vi "Setup Path.vi"(0 "Path in":refnum<class "Path.lvclass">, 5 "TSM Context":T1, 7 "Path Callback References in":refnum<vi>[](array[refnum]), 11 "error in":errorcluster) -> (4 "Path out":refnum<class "Path.lvclass">, 15 "error out":errorcluster)   [LabVIEW 2023, in "RFFixtureCharact.Public.lvlib"]
uses:
  RFFixtureCharact.Public.lvlib
  Common/Base Classes/Path/Path.lvclass
  <vilib>/NI_TestStand_SemiconductorModule/NI_TestStand_Semiconductor_Module.lvlibp/PinMap/General/SemiconductorModuleContext.ctl
  Common/RFCalAndFixtureCharact.Common.lvlib
  <vilib>/NI_TestStand_SemiconductorModule/NI_TestStand_Semiconductor_Module.lvlibp
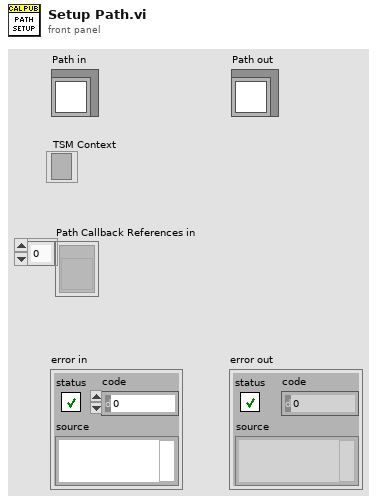
[diagram p1: front panel]
types:
  T1 = typedef "NI_TestStand_Semiconductor_Module.lvlibp/SemiconductorModuleContext.ctl" = refnum<k7>
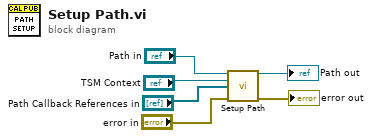
[diagram p0: block diagram]
diagram:
  n1 = call "Setup Path.vi"("Path in"="Path in", "TSM Context"="TSM Context", "Path Callbacks"="Path Callback References in", "error in"="error in") -> ("Path out"=→"Path out":refnum<class "Path.lvclass">, "error out"=→"error out":errorcluster)  [unwired: 10 in]
